vi "Region-det-main_backup.vi"(7 "JSON information string":string, 8 "error in (no error)":errorcluster, 10 "State":dbl[](array[numeric]), 11 "JSON string for Q matrices":string) -> (0 "error out":errorcluster, 2 "Region":dbl)   [LabVIEW 2016]
uses:
  <vilib>/Analysis/baseanly.llb/Real A x B.vi
  <vilib>/Analysis/Matrix/Numeric/Conversions/Array To Matrix - RA.vi
  <vilib>/Analysis/NI_AALBase.lvlib
  <vilib>/Analysis/Matrix/NI_Matrix.lvlib
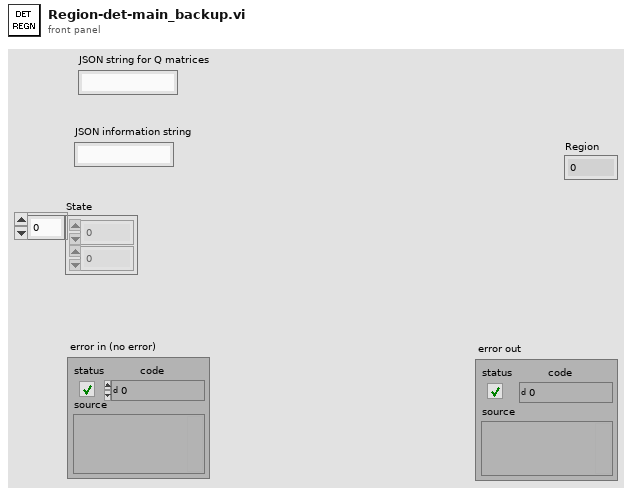
[diagram p1: front panel]
types:
  T1 = typedef "NI_Matrix.lvlib/RealMatrix.ctl" = dbl[][]
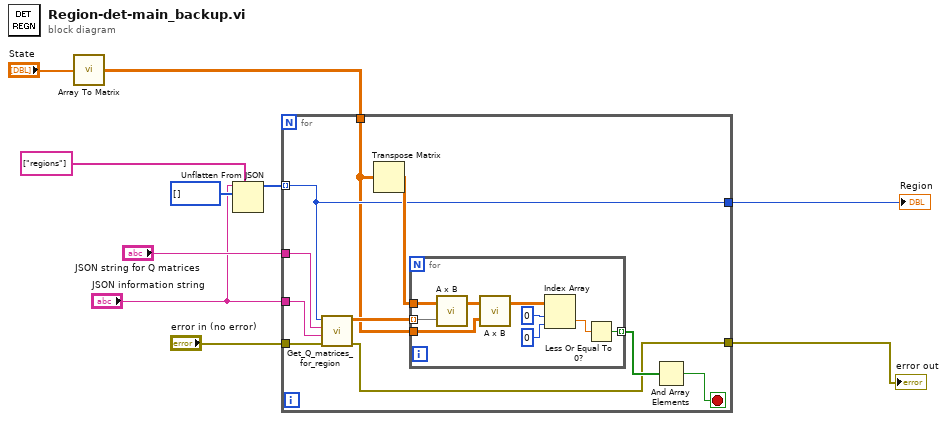
[diagram p0: block diagram]
diagram:
  n1 = call-poly <vilib>:"Array To Matrix.vi"("Real 1D Array"="State") -> ("Real Matrix (Column Vector)"=w1:T1)
  n2 = Unflatten From JSON(path=string[] ["regions"], JSON string="JSON information string", type and defaults=i32[] []) -> (value=w8:i32[])  [unwired: 4 in, 1 out]
  n3 = for {
    tunnel: w8 -> [w13] mode=indexing
    tunnel: "JSON string for Q matrices" -> [w18]
    tunnel: "error in (no error)" -> [w20]
    tunnel: "JSON information string" -> [w19]
    tunnel: [w13] -> w4
    tunnel: [w12] -> w3
    tunnel: w1 -> [w11]
    stop <- w14 stop-if-true
    n4 = call "Get_Q_matrices_for_region.vi"("error in (no error)"=w20, "Q region size JSON string"=w19, "Q matrix JSON string"=w18, "Region"=w13) -> ("error out"=w12:errorcluster, "Q Matrices"=w17:dbl[][][])  [unwired: 6 in]
    n5 = Transpose Matrix(1:w11) -> (0:w16:T1)
    n6 = for {
      tunnel: w17 -> [w28] mode=indexing
      tunnel: w16 -> [w29]
      tunnel: w11 -> [w27]
      tunnel: [w21] -> w15 mode=indexing
      n7 = call-poly <vilib>:"A x B.vi"("B"=w28, "A"=w29) -> ("A x B"=w26:T1)  [unwired: 1 out]
      n8 = call-poly <vilib>:"A x B.vi"("B"=w27, "A"=w26) -> ("A x B"=w25:T1)  [unwired: 1 out]
      n9 = Index Array(array=w25, index (row)=0, index (col)=0) -> (element=w22:dbl)
      n10 = Less Or Equal To 0?(x=w22) -> (x <= 0?=w21:bool)
    }
    n11 = And Array Elements(Boolean array=w15) -> (logical AND=w14:bool)
  }
  "Region" <- w4
  "error out" <- w3
